vi "Byte Buffer.Buffer Subset.Set.vi"(8 "error in (no error)":errorcluster, 9 "offset (0)":u64, 10 "string in":string, 11 "Byte Buffer in":refnum<class "Byte Buffer.lvclass">) -> (0 "error out":errorcluster, 2 "string out":string, 3 "Byte Buffer out":refnum<class "Byte Buffer.lvclass">)   [LabVIEW 2016, in "VeriStand Data.lvlib" / "Byte Buffer.lvclass"]
uses:
  Byte Buffer.lvclass
  Byte Buffer.lvclass/Byte Buffer.ctl
  Memory Management/Memory Management.Handle Return.vi
  VeriStand Data.lvlib
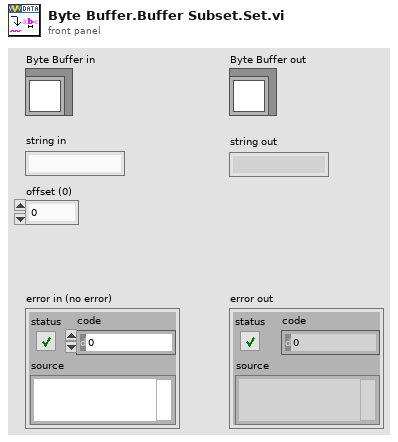
[diagram p1: front panel]
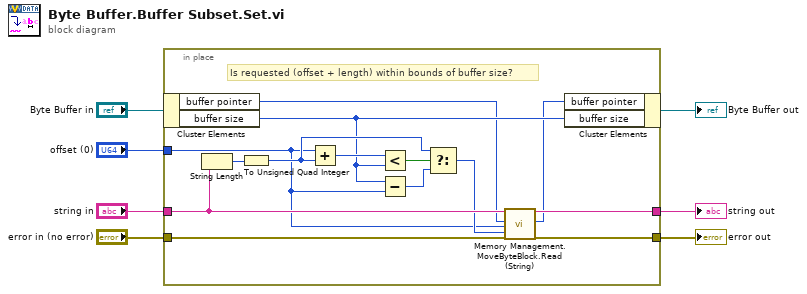
[diagram p0: block diagram]
diagram:
  n1 = in-place {
    in-place-border: "error in (no error)" -> [w14]
    in-place-border: "string in" -> [w12]
    in-place-border: "offset (0)" -> [w10]
    in-place-border: [w15] -> w3
    in-place-border: [w13] -> w2
    # "Is requested (offset + length) within bounds of buffer size?"
    n2 = in-place-cluster #1("Byte Buffer in") -> ("buffer pointer"=w9:u64, "buffer size"=w17:u64)
    n3 = String Length(string=w12) -> (length=w20:i32)
    n4 = To Unsigned Quad Integer(1:w20) -> (0:w18:u64)
    n5 = Add(x=w10, y=w18) -> (x+y=w19:u64)
    n6 = Less?(x=w19, y=w17) -> (x < y?=w21:bool)
    n7 = Subtract(x=w17, y=w10) -> (x-y=w16:u64)
    n8 = Select(t=w18, s=w21, f=w16) -> (s? t:f=w11:u64)
    n9 = call "Memory Management.MoveByteBlock.Read (String).vi"("src in"=w12, "dst ptr in"=w9, "dst offset (0)"=w10, "size"=w11, "error in (no error)"=w14) -> ("src out"=w13:string, "dst ptr out"=w8:u64, "error out"=w15:errorcluster)  [unwired: 9 in, 3 out]
    n10 = in-place-cluster #1("buffer pointer"=w8, "buffer size"=w17) -> (→"Byte Buffer out":refnum<class "Byte Buffer.lvclass">)
  }
  "error out" <- w3
  "string out" <- w2
